vi "BurstModeCompleteRoutedMessage_Send.vi"(8 "error in (no error)":errorcluster, 10 "BurstModeComplete":T1, 11 "Qbus in":refnum<class "Qbus.lvclass">) -> (0 "error out":errorcluster, 3 "Qbus out":refnum<class "Qbus.lvclass">)   [LabVIEW 2017, in "BurstMode.lvlib"]
uses:
  <vilib>/addons/InsightCM/Devices/Shared/Cms/CmsBurstMode/BurstMode.lvlib
  <vilib>/addons/Qbus/Qbus.lvclass
  <vilib>/addons/InsightCM/Devices/Shared/Cms/CmsBurstMode/controls/BurstModeComplete.ctl
  <vilib>/addons/InsightCM/Devices/Shared/Common/Controller/Controller.lvlib
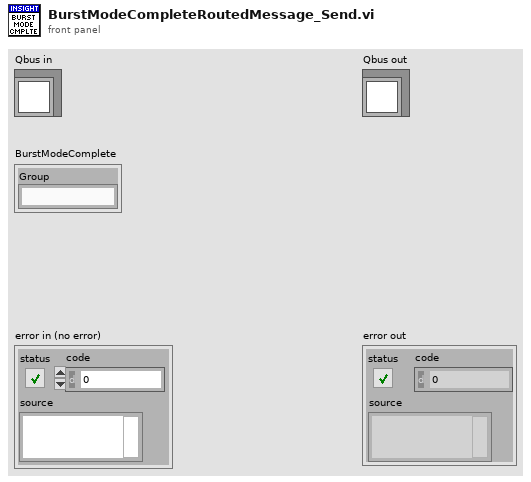
[diagram p1: front panel]
types:
  T1 = typedef "BurstMode.lvlib/BurstModeComplete.ctl" = cluster{"Group":string}
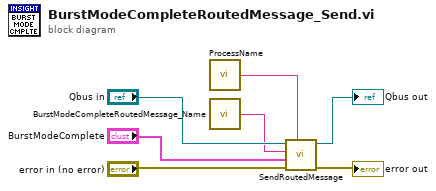
[diagram p0: block diagram]
diagram:
  n1 = call <vilib>:"ProcessName.vi"() -> ("ProcessName"=w1:string)  [unwired: 5 in]
  n2 = call <vilib>:"BurstModeCompleteRoutedMessage_Name.vi"() -> ("message name"=w2:string)  [unwired: 5 in]
  n3 = call <vilib>:"SendRoutedMessage.vi"("listener process"=w1, "error in (no error)"="error in (no error)", "message value"="BurstModeComplete", "message name"=w2, "Qbus in"="Qbus in") -> ("error in (no error)"=→"error out":errorcluster, "Qbus out"=→"Qbus out":refnum<class "Qbus.lvclass">)  [unwired: 5 in]
